vi "enable multiple controls.vi"(8 "error in (no error)":errorcluster, 10 "enabled? (T)":bool=TRUE, 11 "controls in":refnum<vi>[](array[refnum])) -> (0 "error out":errorcluster, 2 "enabled out":bool=TRUE, 3 "controls out":refnum<vi>[](array[refnum]))   [LabVIEW 2014, in "Shared Memory editor node.lvclass"]
uses:
  Shared Memory editor node.lvclass
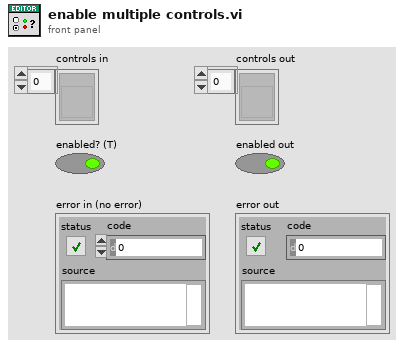
[diagram p1: front panel]
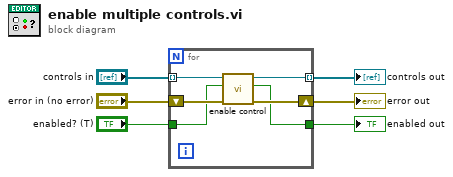
[diagram p0: block diagram]
diagram:
  n1 = for {
    shift-right: [w11] -> w3
    shift-left: "error in (no error)" -> [w12]
    tunnel: "controls in" -> [w10] mode=indexing
    tunnel: [w9] -> w4 mode=indexing
    tunnel: "enabled? (T)" -> [w8]
    tunnel: [w7] -> w1
    n2 = call "enable control.vi"("error in (no error)"=w12, "enabled? (T)"=w8, "control in"=w10) -> ("error out"=w11:errorcluster, "enabled out"=w7:bool, "control out"=w9:refnum<vi>)  [unwired: 6 in]
  }
  "error out" <- w3
  "enabled out" <- w1
  "controls out" <- w4
